vi "Part 2.vi"(11 "Input":string) -> (3 "output":i64)   [LabVIEW 2021]
uses:
  <userlib>/_OpenG.lib/string/string.llb/Convert EOLs (String)__ogtk.vi
panel:
  in  "stop":bool
  out "Array":string[][](array[string])
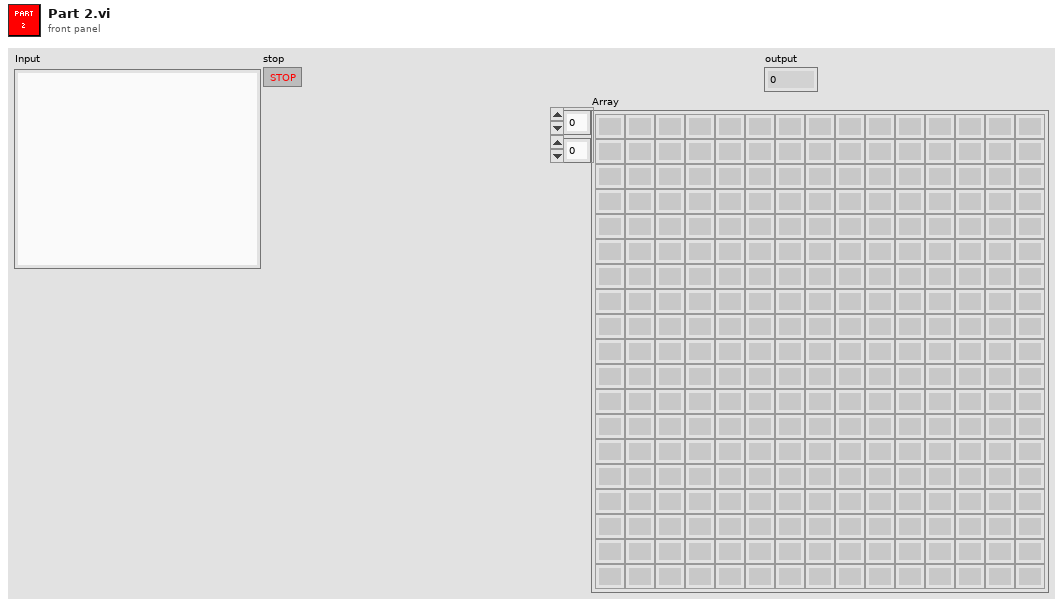
[diagram p1: front panel]
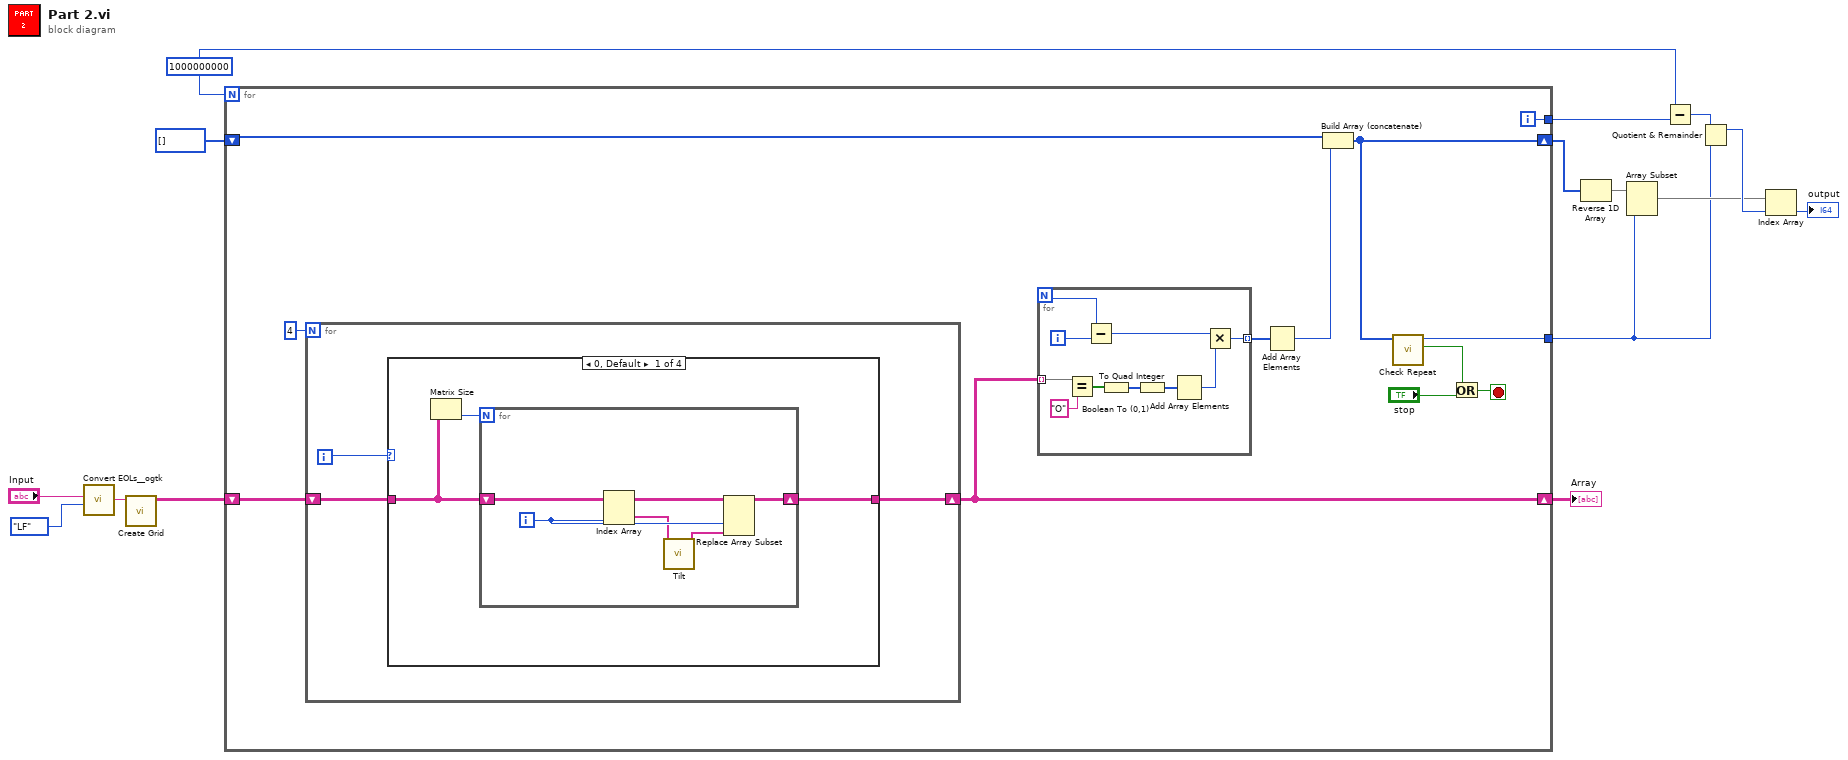
[diagram p0: block diagram]
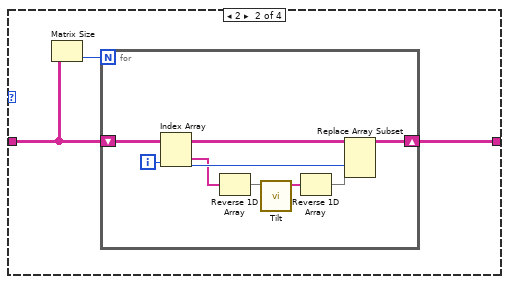
[diagram p2: hidden frame]
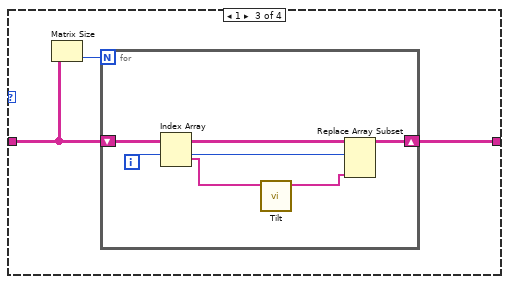
[diagram p3: hidden frame]
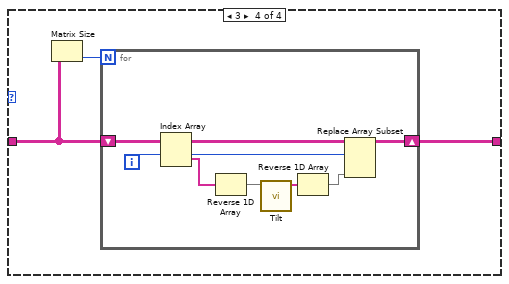
[diagram p4: hidden frame]
diagram:
  w3 = 1000000000
  n1 = call-poly <userlib>:"Convert EOLs__ogtk.vi"("Convert to:"=enum16{"CR", "LF", "CRLF"}."LF", "String in"="Input") -> ("String out"=w13:string)  [unwired: 9 in]
  n2 = call "Create Grid.vi"("String"=w13) -> ("Array"=w12:string[][])  [unwired: 10 in]
  n3 = for {
    N: w3 -> [_]
    shift-right: [w25] -> w11
    shift-left: w12 -> [w26]
    shift-right: [w19] -> w6
    shift-left: i32[] [] -> [w23]
    tunnel: [w18] -> w1
    tunnel: [w16] -> w5
    i -> [w16]
    stop <- w20 stop-if-true
    n4 = for {
      N: 4 -> [_]
      shift-right: [w29] -> w25
      shift-left: w26 -> [w30]
      i -> [w28]
      n5 = case shown="0, Default" w28 {
        tunnel: w30 -> [w32 w40 w50 w58]
        tunnel: [w31 w39 w49 w57] -> w29
        frame 0, Default {
          n6 = Matrix Size(0:w32) -> (2:w33:i32)  [unwired: 1 out]
          n7 = for {
            N: w33 -> [_]
            shift-right: [w37] -> w31
            shift-left: w32 -> [w38]
            i -> [w36]
            n8 = Index Array(array=w38, index (col)=w36) -> (element=w34:string[])  [unwired: 1 in]
            n9 = call "Tilt.vi"("Array in"=w34) -> ("Array out"=w35:string[])  [unwired: 10 in]
            n10 = Replace Array Subset(array=w38, new element=w35, index (col)=w36) -> (w37:string[][])  [unwired: 1 in]
          }
        }
        frame 2 {
          n11 = Matrix Size(0:w40) -> (2:w41:i32)  [unwired: 1 out]
          n12 = for {
            N: w41 -> [_]
            shift-right: [w47] -> w39
            shift-left: w40 -> [w48]
            i -> [w46]
            n13 = Index Array(array=w48, index (col)=w46) -> (element=w45:string[])  [unwired: 1 in]
            n14 = Reverse 1D Array(array=w45) -> (reversed array=w43:string[])
            n15 = call "Tilt.vi"("Array in"=w43) -> ("Array out"=w44:string[])  [unwired: 10 in]
            n16 = Reverse 1D Array(array=w44) -> (reversed array=w42:string[])
            n17 = Replace Array Subset(array=w48, new element=w42, index (col)=w46) -> (w47:string[][])  [unwired: 1 in]
          }
        }
        frame 1 {
          n18 = Matrix Size(0:w50) -> (2:w51:i32)  [unwired: 1 out]
          n19 = for {
            N: w51 -> [_]
            shift-right: [w55] -> w49
            shift-left: w50 -> [w56]
            i -> [w52]
            n20 = Index Array(array=w56, index (row)=w52) -> (element=w54:string[])  [unwired: 1 in]
            n21 = call "Tilt.vi"("Array in"=w54) -> ("Array out"=w53:string[])  [unwired: 10 in]
            n22 = Replace Array Subset(array=w56, new element=w53, index (row)=w52) -> (w55:string[][])  [unwired: 1 in]
          }
        }
        frame 3 {
          n23 = Matrix Size(0:w58) -> (2:w59:i32)  [unwired: 1 out]
          n24 = for {
            N: w59 -> [_]
            shift-right: [w65] -> w57
            shift-left: w58 -> [w66]
            i -> [w62]
            n25 = Index Array(array=w66, index (row)=w62) -> (element=w64:string[])  [unwired: 1 in]
            n26 = Reverse 1D Array(array=w64) -> (reversed array=w61:string[])
            n27 = call "Tilt.vi"("Array in"=w61) -> ("Array out"=w63:string[])  [unwired: 10 in]
            n28 = Reverse 1D Array(array=w63) -> (reversed array=w60:string[])
            n29 = Replace Array Subset(array=w66, new element=w60, index (row)=w62) -> (w65:string[][])  [unwired: 1 in]
          }
        }
      }
    }
    n30 = for {
      N -> [w75]
      tunnel: w25 -> [w73] mode=indexing
      tunnel: [w68] -> w27 mode=indexing
      i -> [w76]
      n31 = Equal?(x=w73, y="O") -> (x = y?=w71:bool[])
      n32 = Subtract(x=w75, y=w76) -> (x-y=w74:i32)
      n33 = Boolean To (0,1)(Boolean=w71) -> (0, 1=w70:i16[])
      n34 = To Quad Integer(1:w70) -> (0:w67:i64[])
      n35 = Add Array Elements(numeric array=w67) -> (sum=w69:i64)
      n36 = Multiply(x=w74, y=w69) -> (x*y=w68:i64)
    }
    n37 = Add Array Elements(numeric array=w27) -> (sum=w22:i64)
    n38 = Build Array (concatenate)(w23, w22) -> (w19:i64[])
    n39 = call "Check Repeat.vi"("Array"=w19) -> ("Repeat?"=w17:bool, "Pattern Length"=w18:i32)  [unwired: 9 in]
    n40 = Or(x=w17, y="stop") -> (x .or. y?=w20:bool)
  }
  "Array" <- w11
  n41 = Reverse 1D Array(array=w6) -> (reversed array=w9:i64[])
  n42 = Array Subset(array=w9, length=w1) -> (w2:i64[])  [unwired: 1 in]
  n43 = Subtract(x=w3, y=w5) -> (x-y=w4:i32)
  n44 = Quotient & Remainder(x=w4, y=w1) -> (x-y*floor(x/y)=w8:i32)  [unwired: 1 out]
  n45 = Index Array(array=w2, index=w8) -> (element=→"output":i64)
